vi "Instrument fgv uno.vi"(7 "Enum":T1(ring), 8 "error in (no error) 2":errorcluster, 10 "WriteCC1":string[](array[string])=[""], 11 "INPUT":T2) -> (0 "error":errorcluster, 2 "WriteCC1":string[](array[string]), 3 "output":T2)   [LabVIEW 2025]
uses:
  cf2ff1be-2106-4981-a75b-2e942dcf7eff.vi
  <vilib>/Instr/_visa.llb/VISA Configure Serial Port (Instr).vi
panel:
  out "read buffer":string
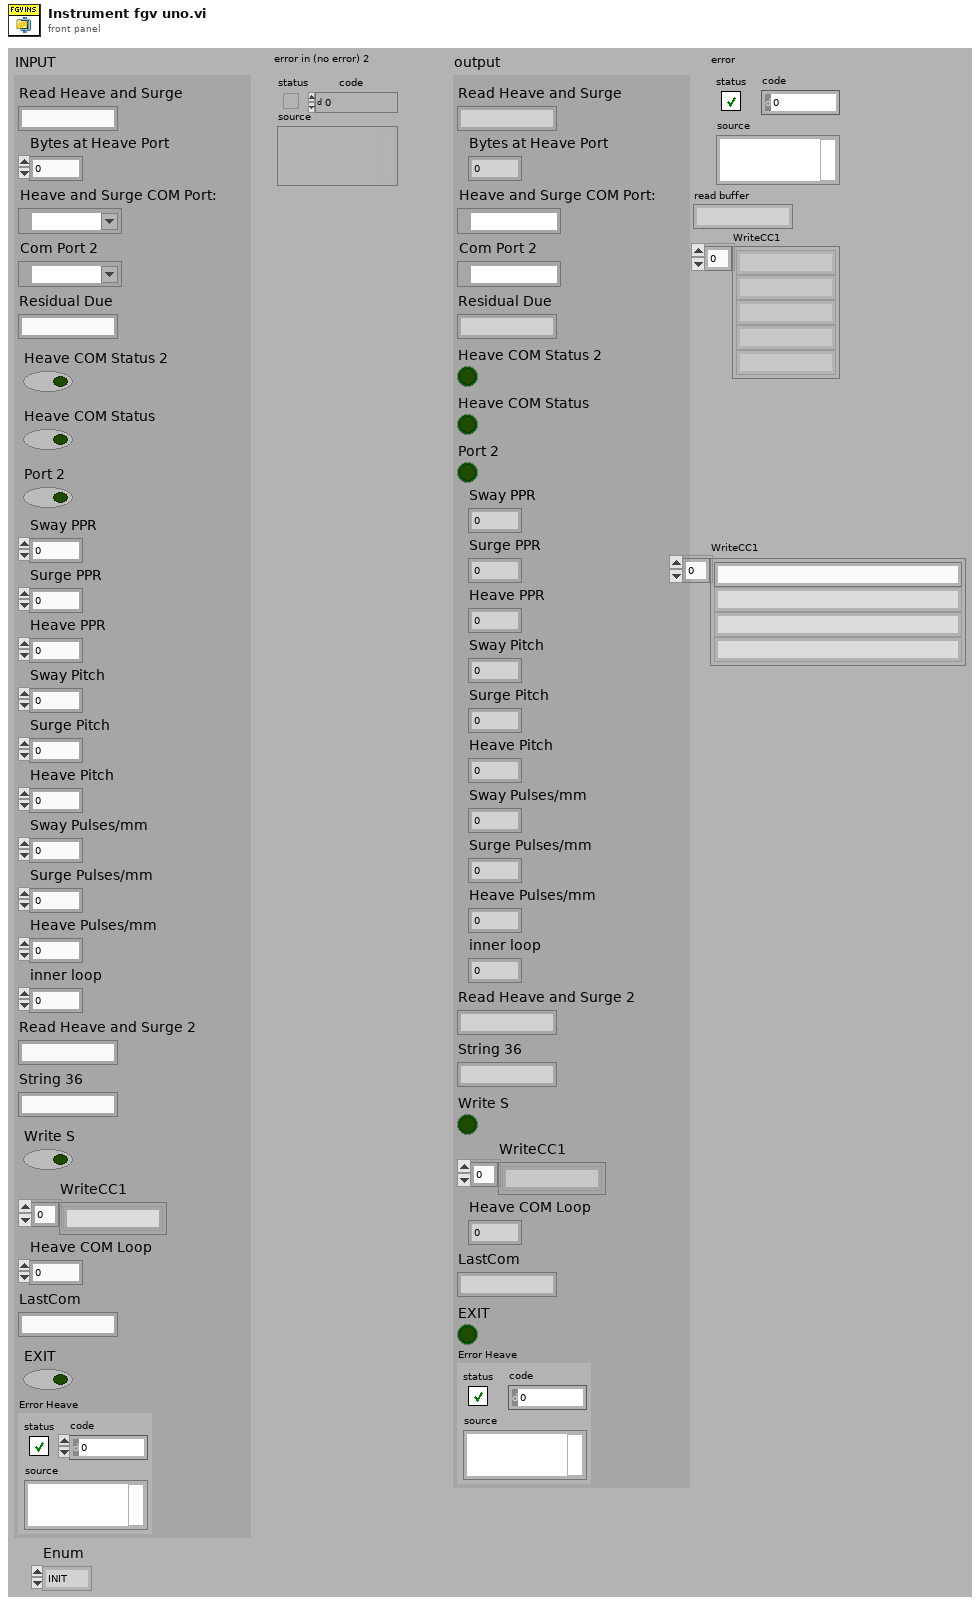
[diagram p1: front panel]
types:
  T1 = enum16{"INIT", "READ", "MANUAL WRITE", "WRITE", "CLOSE", "ERROR INIT"}
  T2 = cluster{"Read Heave and Surge":string, "Bytes at Heave Port":dbl, "Heave and Surge COM Port:":refnum<visa-resource-name>, "Com Port 2":refnum<visa-resource-name>, "Residual Due":string, "Heave COM Status 2":bool, "Heave COM Status":bool, "Port 2":bool, "Sway PPR":dbl, "Surge PPR":dbl, "Heave PPR":dbl, "Sway Pitch":dbl, "Surge Pitch":dbl, "Heave Pitch":dbl, "Sway Pulses/mm":dbl, "Surge Pulses/mm":dbl, "Heave Pulses/mm":dbl, "inner loop":dbl, "Read Heave and Surge 2":string, "String 36":string, "Write S":bool, "WriteCC1":string[], "Heave COM Loop":i32, "LastCom":string, "EXIT":bool, "Error Heave":errorcluster}
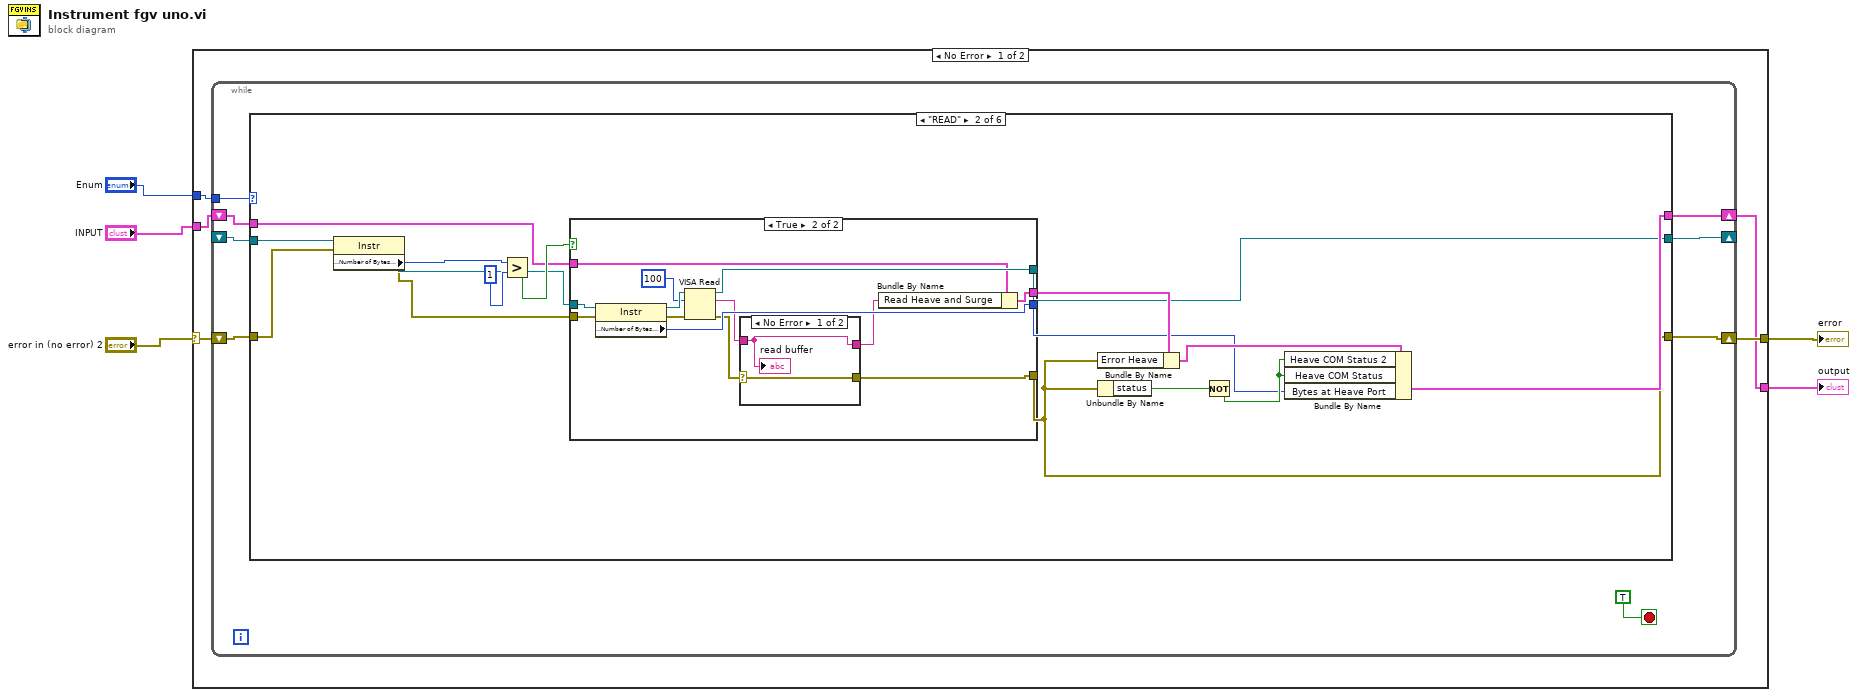
[diagram p0: block diagram]
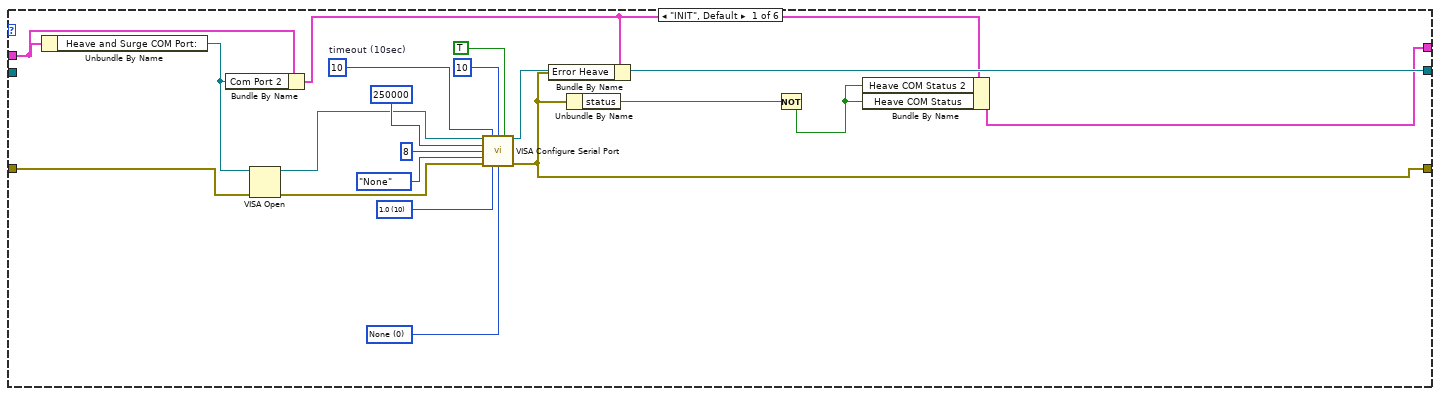
[diagram p2: hidden frame]
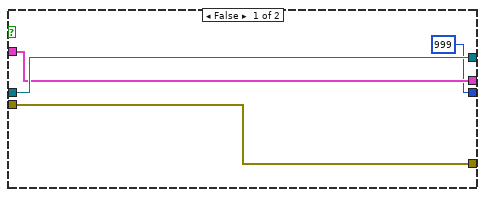
[diagram p3: hidden frame]
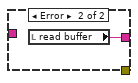
[diagram p4: hidden frame]
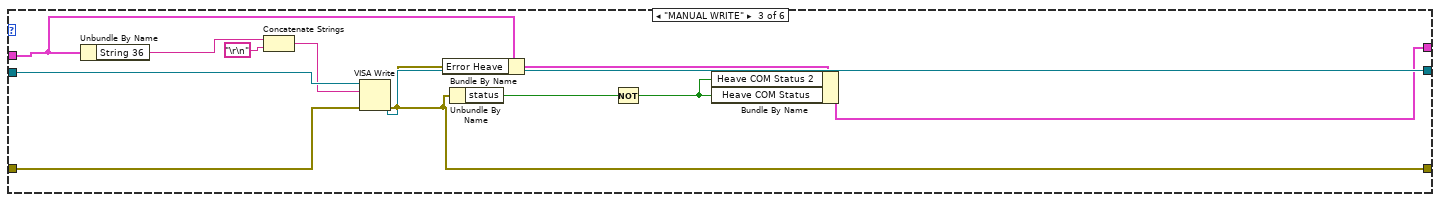
[diagram p5: hidden frame]
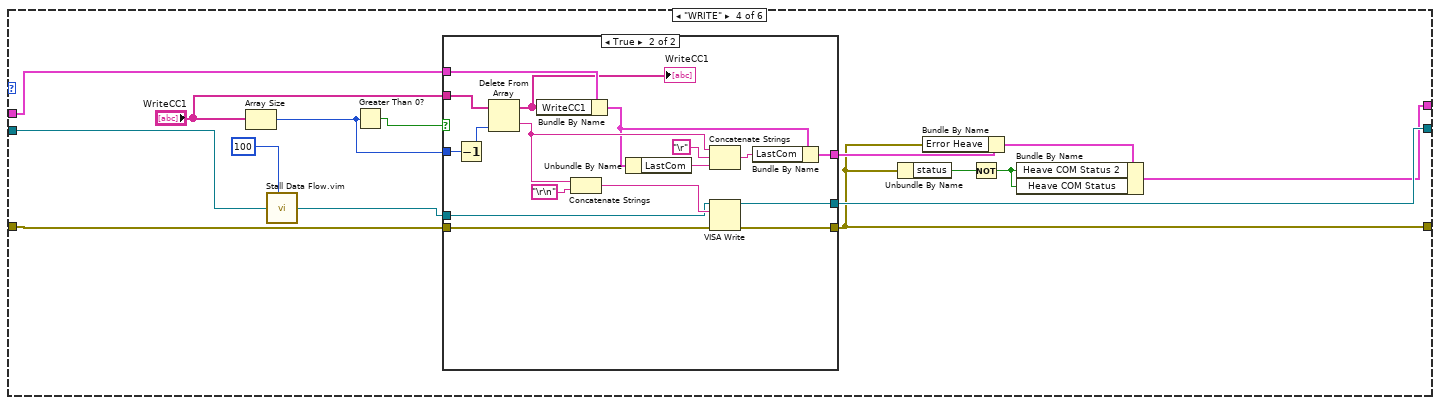
[diagram p6: hidden frame]
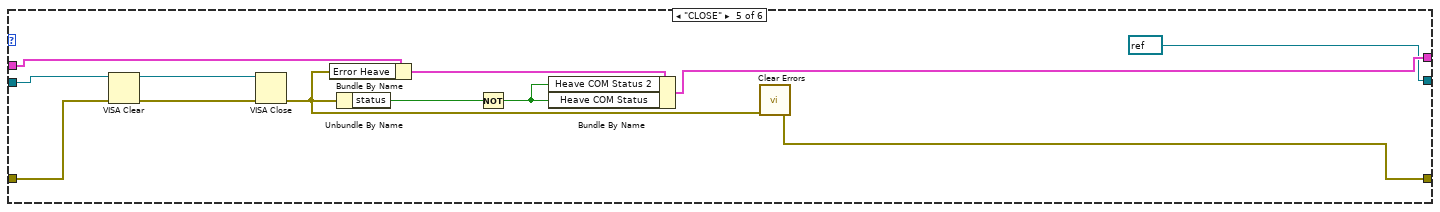
[diagram p8: hidden frame]
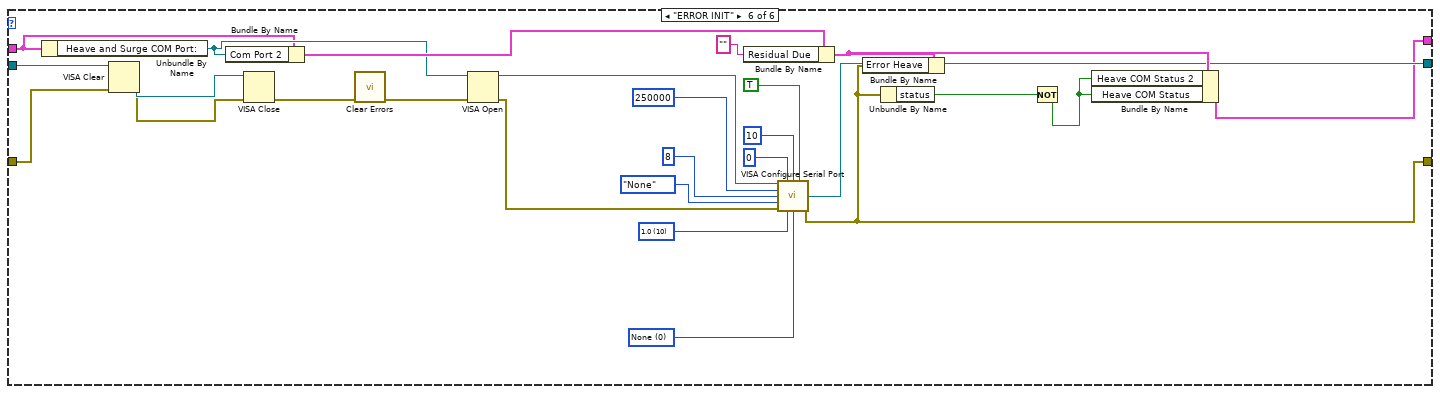
[diagram p9: hidden frame]
diagram:
  n1 = case shown="No Error" "error in (no error) 2" {
    selector: "error in (no error) 2" -> [w9 w159]
    tunnel: [w10 w159] -> w2
    tunnel: "Enum" -> [w8 _]
    tunnel: "INPUT" -> [w7 w160]
    tunnel: [w6 w160] -> w5
    frame No Error {
      n2 = while {
        tunnel: w8 -> [w17]
        shift-right: [w13] -> w10
        shift-left: w9 -> [w14]
        shift-right: [w16] -> w6
        shift-left: w7 -> [w15]
        shift-right: [w12] -> _
        shift-left: _ -> [w11]
        stop <- TRUE ("stop 3") stop-if-true
        n3 = case shown="\"READ\"" w17 {
          tunnel: [w29 w42 w77 w93 w122 w136] -> w16
          tunnel: w15 -> [w25 w46 w79 w96 w123 w140]
          tunnel: w14 -> [w26 w53 w83 w98 w130 w155]
          tunnel: [w22 w39 w78 w92 w128 w138] -> w13
          tunnel: [w30 w41 w84 w97 refnum<visa-resource-name> refnum ("duplicate VISA resource name") w137] -> w12
          tunnel: w11 -> [_ w52 w85 w88 w129 w154]
          frame "INIT", Default {
            w37 = u16 0 items=["None", "XON/XOFF", "RTS/CTS", "XON/XOFF & RTS/CTS", "DTR/DSR", "XON/XOFF & DTR/DSR"] ("flow control (0:none)  2")
            w35 = u16 10 items=["1.0"=10, "1.5"=15, "2.0"=20] ("stop bits 2")
            w33 = u32 10  # timeout (10sec)
            n4 = Unbundle By Name(w25) -> ("Heave and Surge COM Port:"=w23:refnum<visa-resource-name>)
            n5 = Bundle By Name(cluster=w25, "Com Port 2"=w23) -> (w24:T2)
            n6 = VISA Open(error in (no error)=w26, VISA resource name=w23) -> (VISA resource name=w31:refnum<visa-resource-name>, error out=w32:errorcluster)  [unwired: 3 in]
            n7 = call-poly "VISA Configure Serial Port"("VISA resource name"=w31, "timeout (10sec)"=w33, "termination char\n(0xA = '\\n' = LF)"=u8 10 ("termination char\n(0xA = '\\n' = LF)"), "Enable Termination\nChar (T)"=TRUE ("Enable Termination\nChar (T)"), "baud rate (9600)"=u32 250000 ("baud rate  2"), "data bits (8)"=u16 8 ("data bits  2"), "parity (0:none)"=enum16{"None", "Odd", "Even", "Mark", "Space"}."None", "error in (no error)"=w32, "stop bits (10: 1 bit)"=w35, "flow control (0:none)"=w37) -> ("VISA resource name out"=w30:refnum<visa-resource-name>, "error out"=w22:errorcluster)  [unwired: 4 in]
            n8 = Bundle By Name(cluster=w24, "Error Heave"=w22) -> ()  [unwired: 1 out]
            n9 = Unbundle By Name(w22) -> ("status"=w28:bool)
            n10 = Not(x=w28) -> (.not. x?=w27:bool)
            n11 = Bundle By Name(cluster=w24, "Heave COM Status 2"=w27, "Heave COM Status"=w27) -> (w29:T2)
          }
          frame "READ" {
            n12 = property class="Instr"(reference=w52, error in=w53) -> (reference out=w48:refnum<visa-resource-name>, error out=w47:errorcluster, "Serial Settings:Number of Bytes at Serial Port"=w51:u32)
            n13 = Greater?(x=w51, y=u32 1) -> (0:w49:bool)
            n14 = case shown="True" w49 {
              tunnel: w48 -> [w57 w68]
              tunnel: w47 -> [w56 w69]
              tunnel: [w56 w60] -> w39
              tunnel: [w57 w70] -> w41
              tunnel: w46 -> [w55 w67]
              tunnel: [w55 w66] -> w45
              tunnel: [u32 999 ("Bytes at Port") w63] -> w38
              frame False {
              }
              frame True {
                n15 = property class="Instr"(reference=w68, error in=w69) -> (reference out=w65:refnum<visa-resource-name>, error out=w64:errorcluster, "Serial Settings:Number of Bytes at Serial Port"=w63:u32)
                n16 = VISA Read(VISA resource name=w65, byte count=u32 100, error in (no error)=w64) -> (VISA resource name out=w70:refnum<visa-resource-name>, read buffer=w59:string, error out=w61:errorcluster)  [unwired: 1 out]
                n17 = case shown="No Error" w61 {
                  selector: w61 -> [w72 _]
                  tunnel: [w72 _] -> w60
                  tunnel: w59 -> [w71 _]
                  tunnel: [w71 w73] -> w58
                  frame No Error {
                    "read buffer" <- w71
                  }
                  frame Error {
                    n18 = local read "read buffer"() -> (w73:string)
                  }
                }
                n19 = Bundle By Name(cluster=w67, "Read Heave and Surge"=w58) -> (w66:T2)
              }
            }
            n20 = Bundle By Name(cluster=w45, "Error Heave"=w39) -> (w44:T2)
            n21 = Unbundle By Name(w39) -> ("status"=w43:bool)
            n22 = Not(x=w43) -> (.not. x?=w40:bool)
            n23 = Bundle By Name(cluster=w44, "Heave COM Status 2"=w40, "Heave COM Status"=w40, "Bytes at Heave Port"=w38) -> (w42:T2)
          }
          frame "MANUAL WRITE" {
            n24 = Unbundle By Name(w79) -> ("String 36"=w82:string)
            n25 = Concatenate Strings(w82, "\r\n") -> (w75:string)
            n26 = VISA Write(VISA resource name=w85, write buffer=w75, error in (no error)=w83) -> (VISA resource name out=w84:refnum<visa-resource-name>, error out=w78:errorcluster)  [unwired: 1 out]
            n27 = Bundle By Name(cluster=w79, "Error Heave"=w78) -> (w81:T2)
            n28 = Unbundle By Name(w78) -> ("status"=w80:bool)
            n29 = Not(x=w80) -> (.not. x?=w76:bool)
            n30 = Bundle By Name(cluster=w81, "Heave COM Status 2"=w76, "Heave COM Status"=w76) -> (w77:T2)
          }
          frame "WRITE" {
            n31 = Array Size(array="WriteCC1") -> (size(s)=w100:i32)
            n32 = call "Stall Data Flow.vim"("value in"=w88, "milliseconds to wait"=u32 100) -> ("value out"=w87:refnum<visa-resource-name>)  [unwired: 1 out]
            n33 = Greater Than 0?(x=w100) -> (x > 0?=w99:bool)
            n34 = case shown="True" w99 {
              tunnel: [w103 w114] -> w92
              tunnel: w98 -> [w103 w119]
              tunnel: [w101 w118] -> w97
              tunnel: "WriteCC1" -> [_ w115]
              tunnel: w100 -> [_ w117]
              tunnel: w96 -> [w102 w111]
              tunnel: [w102 w109] -> w95
              tunnel: w87 -> [w101 w105]
              frame False {
              }
              frame True {
                n35 = Decrement(x=w117) -> (x-1=w116:i32)
                n36 = Delete From Array(array=w115, index=w116) -> (deleted portion=w113:string, array with subset deleted=w108:string[])  [unwired: 1 in]
                "WriteCC1" <- w108
                n37 = Bundle By Name(cluster=w111, "WriteCC1"=w108) -> (w104:T2)
                n38 = Concatenate Strings(w113, "\r\n") -> (w107:string)
                n39 = Unbundle By Name(w104) -> ("LastCom"=w110:string)
                n40 = Concatenate Strings(w113, "\r", w110) -> (w112:string)
                n41 = VISA Write(VISA resource name=w105, write buffer=w107, error in (no error)=w119) -> (VISA resource name out=w118:refnum<visa-resource-name>, error out=w114:errorcluster)  [unwired: 1 out]
                n42 = Bundle By Name(cluster=w104, "LastCom"=w112) -> (w109:T2)
              }
            }
            n43 = Unbundle By Name(w92) -> ("status"=w91:bool)
            n44 = Bundle By Name(cluster=w95, "Error Heave"=w92) -> (w94:T2)
            n45 = Not(x=w91) -> (.not. x?=w90:bool)
            n46 = Bundle By Name(cluster=w94, "Heave COM Status 2"=w90, "Heave COM Status"=w90) -> (w93:T2)
          }
          frame "CLOSE" {
            n47 = VISA Clear(VISA resource name=w129, error in (no error)=w130) -> (VISA resource name out=w132:refnum<visa-resource-name>, error out=w131:errorcluster)
            n48 = VISA Close(VISA resource name=w132, error in (no error)=w131) -> (error out=w124:errorcluster)
            n49 = Bundle By Name(cluster=w123, "Error Heave"=w124) -> (w127:T2)
            n50 = Unbundle By Name(w124) -> ("status"=w126:bool)
            n51 = Not(x=w126) -> (.not. x?=w125:bool)
            n52 = Bundle By Name(cluster=w127, "Heave COM Status 2"=w125, "Heave COM Status"=w125) -> (w122:T2)
            n53 = call <vilib>:"Clear Errors.vi"("error in (no error)"=w124) -> ("error out"=w128:errorcluster)  [unwired: 5 in, 1 out]
          }
          frame "ERROR INIT" {
            w152 = u16 0 items=["None", "XON/XOFF", "RTS/CTS", "XON/XOFF & RTS/CTS", "DTR/DSR", "XON/XOFF & DTR/DSR"] ("flow control (0:none)  2")
            w150 = u16 10 items=["1.0"=10, "1.5"=15, "2.0"=20] ("stop bits 2")
            n54 = Unbundle By Name(w140) -> ("Heave and Surge COM Port:"=w141:refnum<visa-resource-name>)
            n55 = VISA Clear(VISA resource name=w154, error in (no error)=w155) -> (VISA resource name out=w158:refnum<visa-resource-name>, error out=w157:errorcluster)
            n56 = Bundle By Name(cluster=w140, "Com Port 2"=w141) -> (w142:T2)
            n57 = VISA Close(VISA resource name=w158, error in (no error)=w157) -> (error out=w156:errorcluster)
            n58 = call <vilib>:"Clear Errors.vi"("error in (no error)"=w156) -> ("error out"=w139:errorcluster)  [unwired: 5 in, 1 out]
            n59 = VISA Open(error in (no error)=w139, VISA resource name=w141) -> (VISA resource name=w146:refnum<visa-resource-name>, error out=w147:errorcluster)  [unwired: 3 in]
            n60 = Bundle By Name(cluster=w142, "Residual Due"="") -> (w145:T2)
            n61 = call-poly "VISA Configure Serial Port"("VISA resource name"=w146, "timeout (10sec)"=u32 0, "termination char\n(0xA = '\\n' = LF)"=u8 10 ("termination char\n(0xA = '\\n' = LF)"), "Enable Termination\nChar (T)"=TRUE ("Enable Termination\nChar (T)"), "baud rate (9600)"=u32 250000 ("baud rate  2"), "data bits (8)"=u16 8 ("data bits  2"), "parity (0:none)"=enum16{"None", "Odd", "Even", "Mark", "Space"}."None", "error in (no error)"=w147, "stop bits (10: 1 bit)"=w150, "flow control (0:none)"=w152) -> ("VISA resource name out"=w137:refnum<visa-resource-name>, "error out"=w138:errorcluster)  [unwired: 4 in]
            n62 = Bundle By Name(cluster=w145, "Error Heave"=w138) -> ()  [unwired: 1 out]
            n63 = Unbundle By Name(w138) -> ("status"=w144:bool)
            n64 = Not(x=w144) -> (.not. x?=w143:bool)
            n65 = Bundle By Name(cluster=w145, "Heave COM Status 2"=w143, "Heave COM Status"=w143) -> (w136:T2)
          }
        }
      }
    }
    frame Error {
    }
  }
  "output" <- w5
  "error" <- w2
